vi "Self Test.vi"(8 "error in":errorcluster, 10 "Board Image":T2, 11 "DA Converter in":refnum<class "DA Converter.lvclass">) -> (0 "error out":errorcluster, 2 "Pass?":T1, 3 "DA Converter out":refnum<class "DA Converter.lvclass">)   [LabVIEW 2023, in "DA Converter.lvclass"]
doc: "Check the image for this component's placement on the board."
uses:
  DA Converter.lvclass
  c:/dev/_r/4/eng/lv-core/lvpostprocessingd/lv_mc_x86_64/dist_i386/examples/Object-Oriented Programming/Board Testing/Object Design/Component/Component.lvclass
  Common/Board Image.ctl
  Common/Pass Fail Boolean.ctl
  Component/Component.lvclass
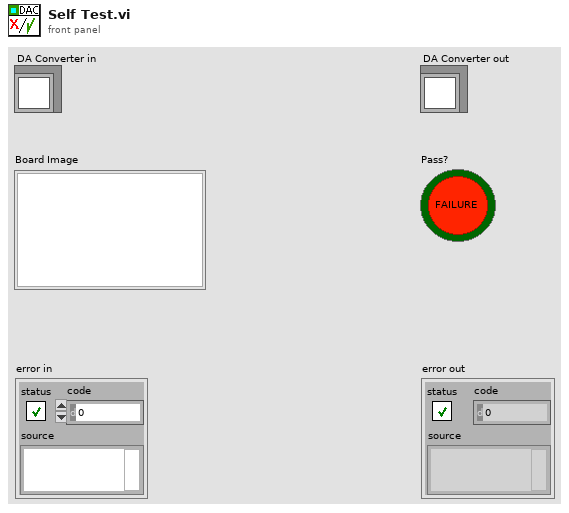
[diagram p1: front panel]
types:
  T1 = typedef "Pass Fail Boolean.ctl" = bool
  T2 = typedef "Board Image.ctl" = picture
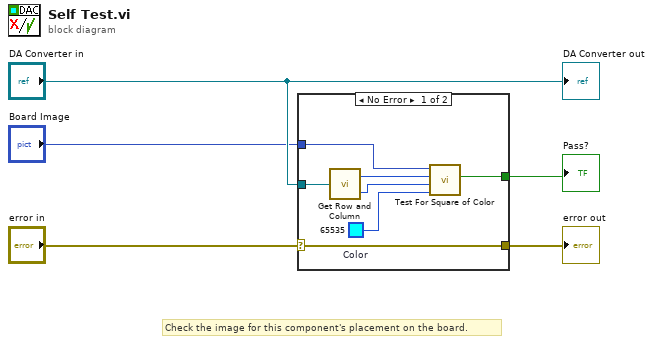
[diagram p0: block diagram]
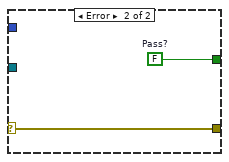
[diagram p2: hidden frame]
diagram:
  # "Check the image for this component's placement on the board."
  n1 = case shown="No Error" "error in" {
    selector: "error in" -> [w10 w14]
    tunnel: [w11 w13] -> w5
    tunnel: [w10 w14] -> w3
    tunnel: "DA Converter in" -> [w9 _]
    tunnel: "Board Image" -> [w6 _]
    frame No Error {
      w12 = u32 65535  # Color
      n2 = call "Get Row and Column.vi"("Component in"=w9) -> ("row"=w8:i16, "column"=w7:i16)
      n3 = call "Test For Square of Color.vi"("color"=w12, "column"=w7, "row"=w8, "board image"=w6) -> ("pass?"=w11:T1)  [unwired: 7 in]
    }
    frame Error {
      w13 = T1 FALSE  # Pass?
    }
  }
  "error out" <- w3
  "Pass?" <- w5
  "DA Converter out" <- "DA Converter in"
